vi "Throw Error - ATO Checkbox Should Be Disabled.vi"(8 "error in":errorcluster) -> (0 "error out":errorcluster)   [LabVIEW 2022 SP3]
doc: "Throws a custom error that indicates that an impossible state was detected.\n\nATO = Add To Owner? checkbox"
panel:
  # "Development\ncontrols/indicators useful for development and testing, but which are not outputs of the VI"
  # "Input\nInputs to the VI"
  # "Output\nOutputs of the VI"
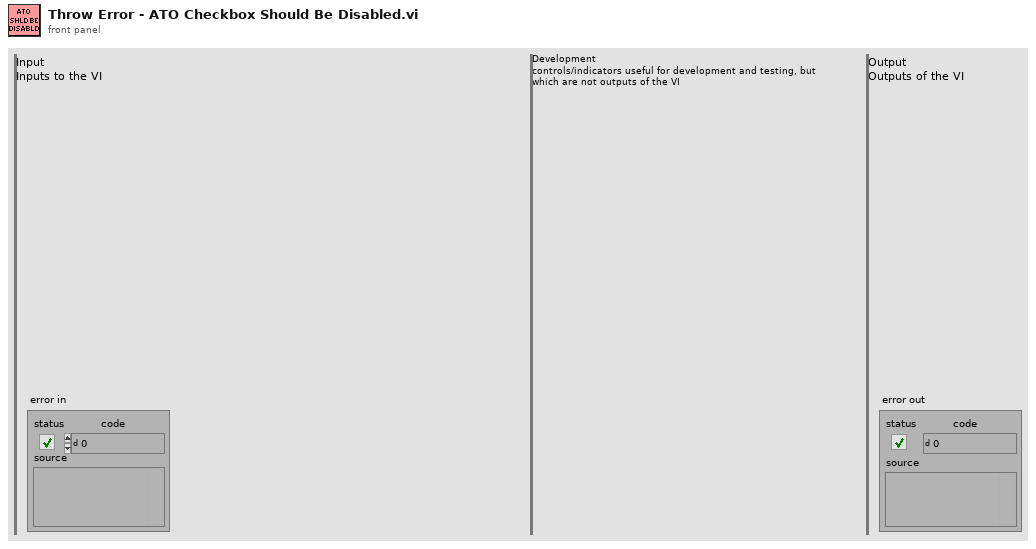
[diagram p1: front panel]
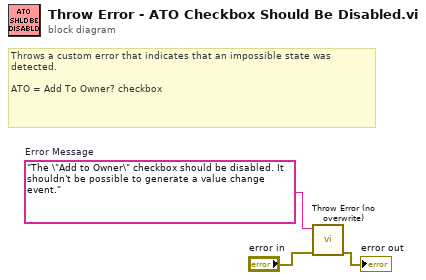
[diagram p0: block diagram]
diagram:
  w3 = "The \"Add to Owner\" checkbox should be disabled. It shouldn't be possible to generate a value change event."  # Error Message
  # "Throws a custom error that indicates that an impossible state was detected.\n\nATO = Add To Owner? checkbox"
  n1 = call "Throw Error (no overwrite).vi"("error in"="error in", "Error Message"=w3) -> ("error out"=→"error out":errorcluster)  [unwired: 9 in]
